vi "Read Menu object array values.vi"(11 "Menu object array":T1 {"Object name" items=["Select one"]}) -> (3 "Values":u16[](array[ring]) items=["Select one"], 4 "Remove object pressed":i32, 5 "Remove object":i32, 6 "Open parameters pressed":i32, 7 "Open parameters for object":i32)   [LabVIEW 2015]
uses:
  Controls/Menu object array.ctl
  Controls/Menu object.ctl
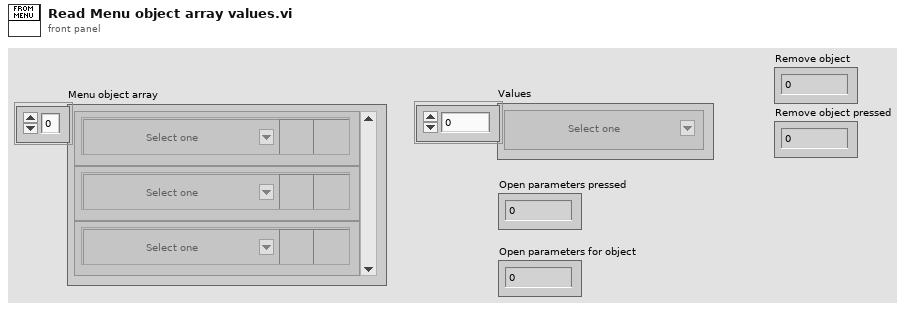
[diagram p1: front panel]
types:
  T1 = typedef "Menu object array.ctl" = T2[]
  T2 = typedef "Menu object.ctl" = cluster{"Object name":u16, "Open parameters":bool, "Remove Button":bool}
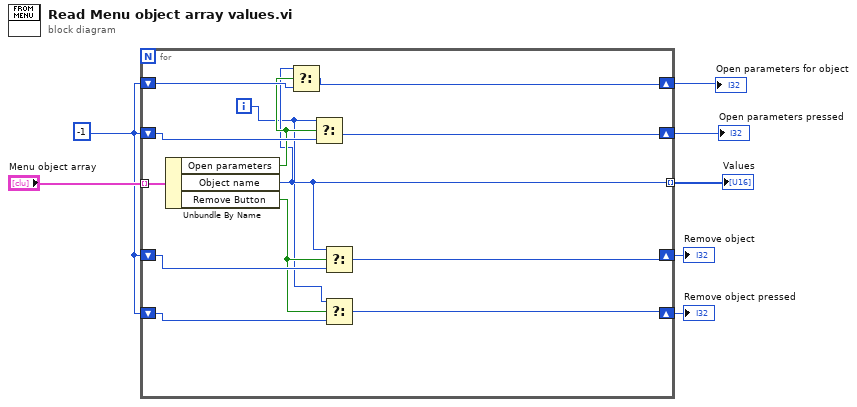
[diagram p0: block diagram]
diagram:
  w3 = -1
  n1 = for {
    tunnel: "Menu object array" -> [w20] mode=indexing
    tunnel: [w9] -> w6 mode=indexing
    shift-right: [w18] -> w5
    shift-left: w3 -> [w19]
    shift-right: [w16] -> w4
    shift-left: w3 -> [w17]
    shift-right: [w14] -> w2
    shift-left: w3 -> [w12]
    shift-right: [w13] -> w1
    shift-left: w3 -> [w11]
    i -> [w8]
    n2 = Unbundle By Name(w20) -> ("Open parameters"=w15:bool, "Object name"=w9:u16, "Remove Button"=w10:bool)
    n3 = Select(t=w9, s=w15, f=w17) -> (s? t:f=w16:i32)
    n4 = Select(t=w8, s=w15, f=w19) -> (s? t:f=w18:i32)
    n5 = Select(t=w9, s=w10, f=w12) -> (s? t:f=w14:i32)
    n6 = Select(t=w8, s=w10, f=w11) -> (s? t:f=w13:i32)
  }
  "Values" <- w6
  "Open parameters pressed" <- w5
  "Open parameters for object" <- w4
  "Remove object" <- w2
  "Remove object pressed" <- w1
